vi "Teleop.vi"(10 "Match Info":T1={"Autonomous Elapsed Seconds"=0.0, "TeleOp Elapsed Seconds"=0.0, "Disabled Elapsed Seconds"=0.0, "Visited Autonomous"=FALSE, "Visited TeleOp"=FALSE, "Visited Disabled"=FALSE, "Autonomous Settings"={"Autonomous Style"=enum."Independent", "VI Refnum"=refnum}}, 11 "Call Context":T2) -> ()   [LabVIEW 2019]
doc: "This VI is called for each TeleOp packet received from the DS where the robot is not disabled. It is often used to read from the joysticks and update I/O or to update setpoints for timed control loops. It should complete and return within 20 milliseconds or it may miss DS packets."
uses:
  <vilib>/Rock Robotics/WPI/DriverStation/WPI_DriverStationDerivedRobotMode.ctl
  <vilib>/Rock Robotics/WPI/DriverStation/WPI_DriverStationMatch Info.ctl
  <vilib>/Rock Robotics/WPI/Utilities/WPI_GetSetVariantRefNum.vi
  <vilib>/Rock Robotics/Network Tables/NT Write Boolean Array.vi
  <vilib>/Rock Robotics/Network Tables/NT Write Numeric Array.vi
  <vilib>/Rock Robotics/Network Tables/NT Read Boolean.vi
  <vilib>/Rock Robotics/Network Tables/NT Read Number.vi
  Downloads/Global 2.vi
  <vilib>/Rock Robotics/Network Tables/NT Write String.vi
  <vilib>/Rock Robotics/WPI/Ultrasonic/WPI_SonarMB1010AnalogRefNum Registry Get.vi
  <vilib>/Rock Robotics/WPI/Ultrasonic/WPI_SonarMB1010AnalogGetRange.vi
  ultraG.vi
  <vilib>/functionblocks/Edge Detection/One Shot Rising with Input/One Shot Rising with Input.vi
  <vilib>/Rock Robotics/WPI/Solenoid/Deprecated/WPI_SolenoidSetBool.vi
  <vilib>/functionblocks/FB Core/FB Core.xnode
  <vilib>/functionblocks/NI_FunctionBlock Libraries.lvlib
panel:
  out "sonic":bool
  out "sensonic":bool
  in  "pegador":bool
  in  "tracao":bool
  in  "roleta":bool
  out "Matched Color Name":string
  out "Matched Color":cluster{"R":dbl, "G":dbl, "B":dbl}
  out "Color":u32(colorbox)
  out "Leitura":cluster{"R":dbl, "G":dbl, "B":dbl}
  out "Sample Slider 0":dbl(slide) scale=0.0..5.0
  out "Sample Boolean 1":bool
  out "Sample Boolean 0":bool
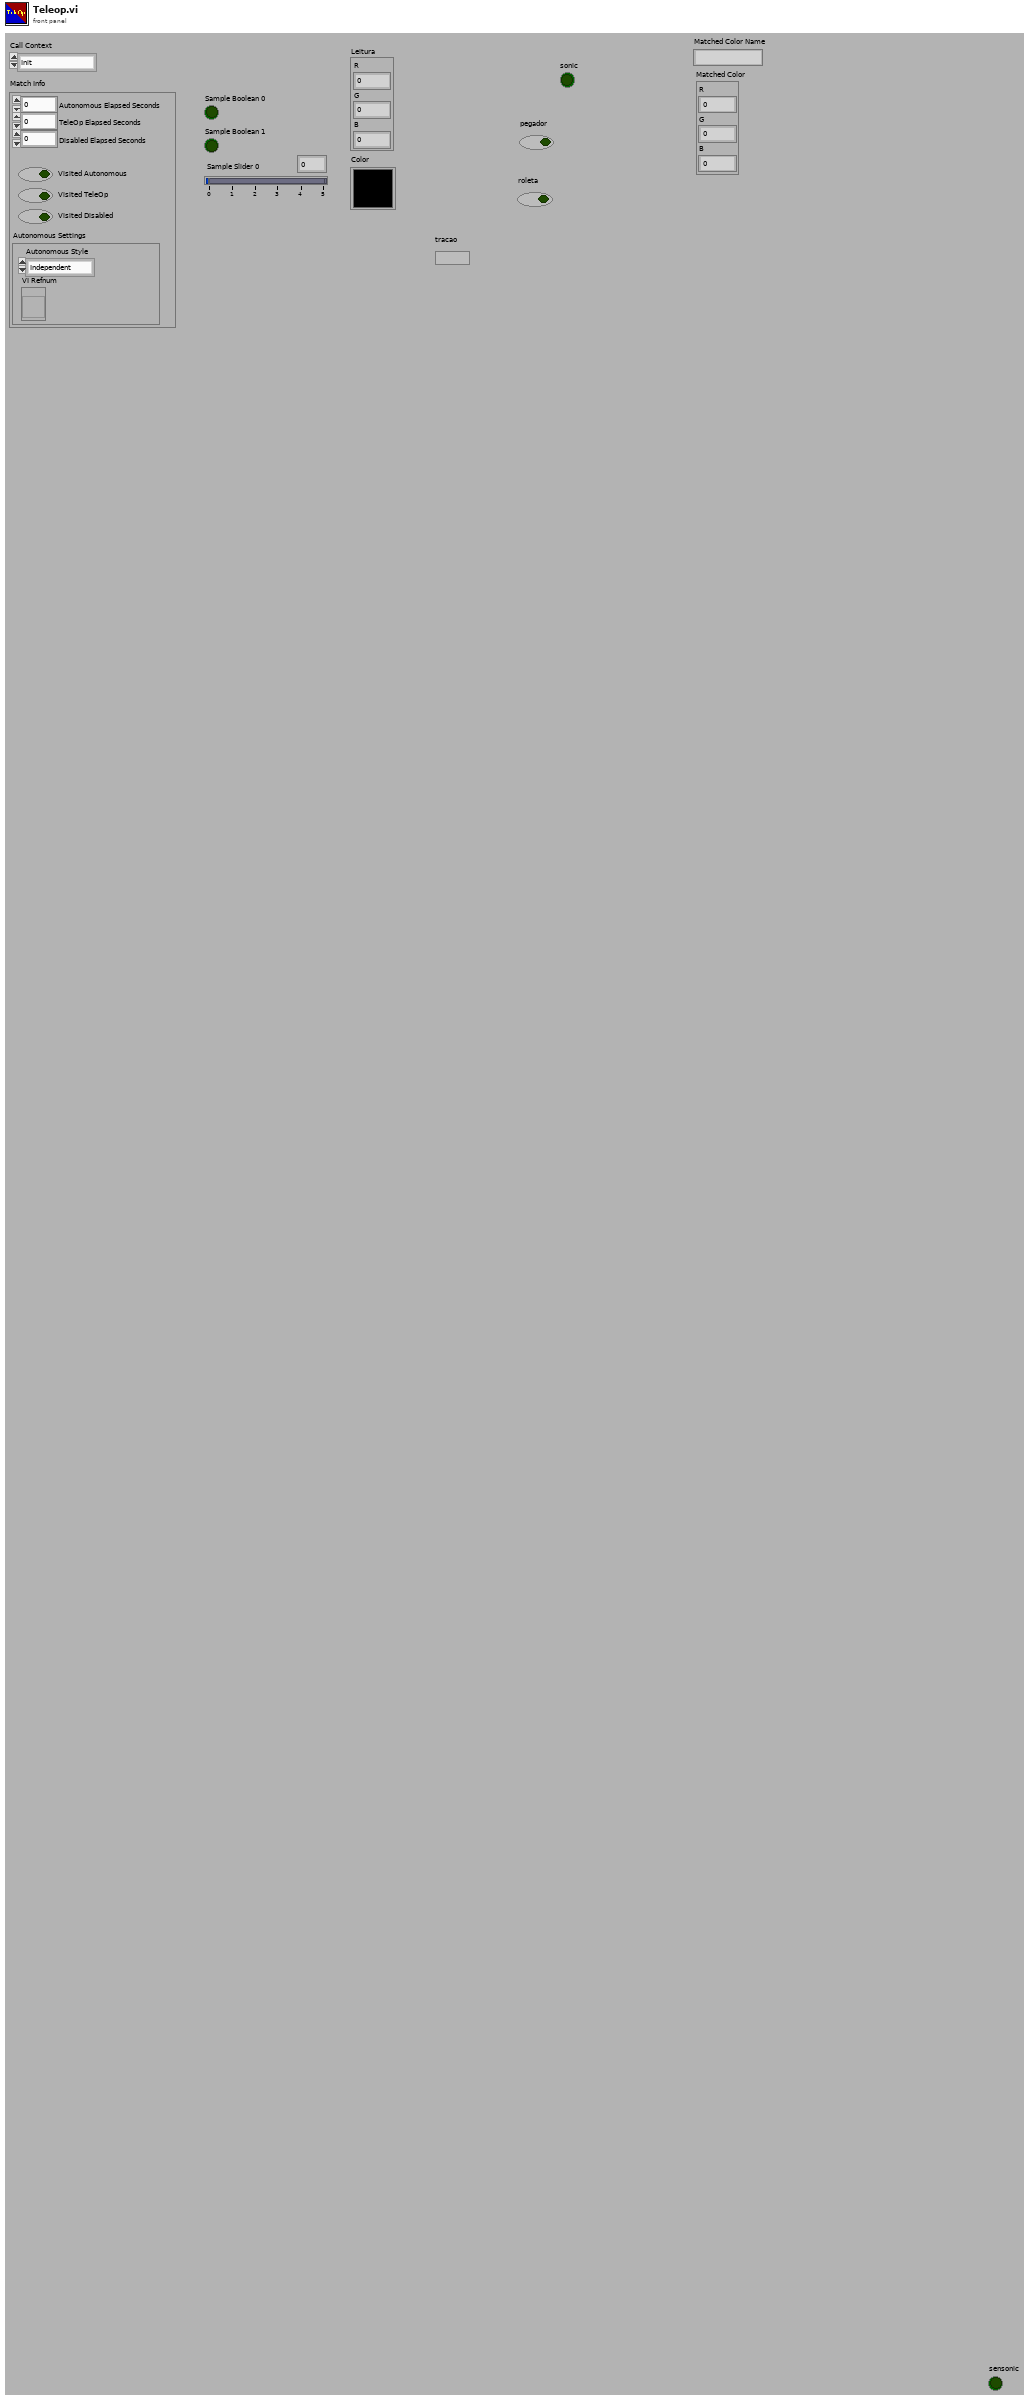
[diagram p1: front panel]
types:
  T1 = typedef "WPI_DriverStationMatch Info.ctl" = cluster{"Autonomous Elapsed Seconds":dbl, "TeleOp Elapsed Seconds":dbl, "Disabled Elapsed Seconds":dbl, "Visited Autonomous":bool, "Visited TeleOp":bool, "Visited Disabled":bool, "Autonomous Settings":cluster{"Autonomous Style":enum16{"Iterative", "Independent"}, "VI Refnum":refnum<vi>}}
  T2 = typedef "WPI_DriverStationDerivedRobotMode.ctl" = enum16{"Init", "Execute", "Stop"}
  T3 = typedef "WPI_MotorControlDeviceRef.ctl" = cluster{"DeviceStatus":errorcluster, "Type":T4, "PWM":cluster{"PWM Channel":T5, "DeadBand":T6}, "CAN":cluster{"Device Number":u8, "SetOutput VI Ref":variant, "GetOutput VI Ref":variant, "Enable VI Ref":variant, "Disable VI Ref":variant, "Data":variant}, "Invert":bool, "DIO PWM":cluster{"PWM \"Enable\" Channel":T5, "DIOChannel":T7, "PWM Rate":dbl}}
  T4 = typedef "WPI_MotorControlType.ctl" = enum16{"PWM", "CAN", "DIO PWM"}
  T5 = typedef "FPGA_DIOPWMChannel.ctl" = enum8{"PWM 0", "PWM 1", "PWM 2", "PWM 3", "PWM 4", "PWM 5", "PWM 6", "PWM 7", "PWM 8", "PWM 9", "PWM MXP 0", "PWM MXP 1", "PWM MXP 2", "PWM MXP 3", "PWM MXP 4", "PWM MXP 5", "PWM MXP 6", "PWM MXP 7", "PWM MXP 8", "PWM MXP 9", "Invalid"}
  T6 = typedef "WPI_PWMDeadband.ctl" = cluster{"Name":string, "maxPositivePwm":i32, "minPositivePwm":i32, "centerPwm":i32, "maxNegativePwm":i32, "minNegativePwm":i32, "angularRange":u16}
  T7 = typedef "FPGA_DIOChannel.ctl" = enum8{"DIO 0", "DIO 1", "DIO 2", "DIO 3", "DIO 4", "DIO 5", "DIO 6", "DIO 7", "DIO 8", "DIO 9", "DIO MXP 0", "DIO MXP 1", "DIO MXP 2", "DIO MXP 3", "DIO MXP 4", "DIO MXP 5", "DIO MXP 6", "DIO MXP 7", "DIO MXP 8", "DIO MXP 9", "DIO MXP 10", "DIO MXP 11", "DIO MXP 12", "DIO MXP 13", "DIO MXP 14", "DIO MXP 15", "SPI Port CS1", "SPI Port CS2", "SPI Port CS3", "SPI Port MISO", "SPI Port MOSI", "Invalid"}
  T8 = typedef "WPI_JoystickDevRef.ctl" = cluster{"Device":T9}
  T9 = typedef "WPI_JoystickDeviceEnum.ctl" = enum16{"USB 0", "USB 1", "USB 2", "USB 3", "USB 4", "USB 5"}
  T10 = cluster{"Axes[0]":dbl, "Axes[1]":dbl, "Axes[2]":dbl, "Axes[3]":dbl, "Axes[4]":dbl, "Axes[5]":dbl, "Axes[6]":dbl, "Axes[7]":dbl, "Axes[8]":dbl}
  T11 = cluster{"Buttons[0]":bool, "Buttons[1]":bool, "Buttons[2]":bool, "Buttons[3]":bool, "Buttons[4]":bool, "Buttons[5]":bool, "Buttons[6]":bool, "Buttons[7]":bool, "Buttons[8]":bool}
  T12 = typedef "WPI_RobotDriveDevRef.ctl" = cluster{"DevStatus":errorcluster, "Motors[]":T3[], "Square Inputs":bool, "Max Output":dbl}
  T13 = typedef "WPI_SolenoidDevRef.ctl" = cluster{"DevStatus":errorcluster, "Pneumatics Control Module":u8, "Forward Solenoid Channel":T14, "Reverse Solenoid Channel":T14}
  T14 = typedef "WPI_SolenoidChannel.ctl" = enum8{"Solenoid 0", "Solenoid 1", "Solenoid 2", "Solenoid 3", "Solenoid 4", "Solenoid 5", "Solenoid 6", "Solenoid 7", "Invalid"}
  T15 = typedef "Color Sensor V3 DevRef.ctl" = cluster{"I2CDevRef":T16}
  T16 = typedef "WPI_I2CDevRef.ctl" = cluster{"DevStatus":errorcluster, "Device Address":u8, "Handle":i32, "I2C Bus":T17}
  T17 = typedef "i2c_bus.ctl" = enum16{"I2C On-Board", "I2C MXP", "Invalid"}
  T18 = typedef "WPI_SonarMB1010AnalogDeviceRef.ctl" = cluster{"AIDeviceRef":T19, "Scaling factor (V/in)":dbl, "Average Bits":u8}
  T19 = typedef "WPI_AnalogChannelDevRef.ctl" = cluster{"DevStatus":errorcluster, "Analog Channel":T20}
  T20 = typedef "FPGA_AIChannel.ctl" = enum8{"AI 0", "AI 1", "AI 2", "AI 3", "AI MXP 0", "AI MXP 1", "AI MXP 2", "AI MXP 3", "Invalid"}
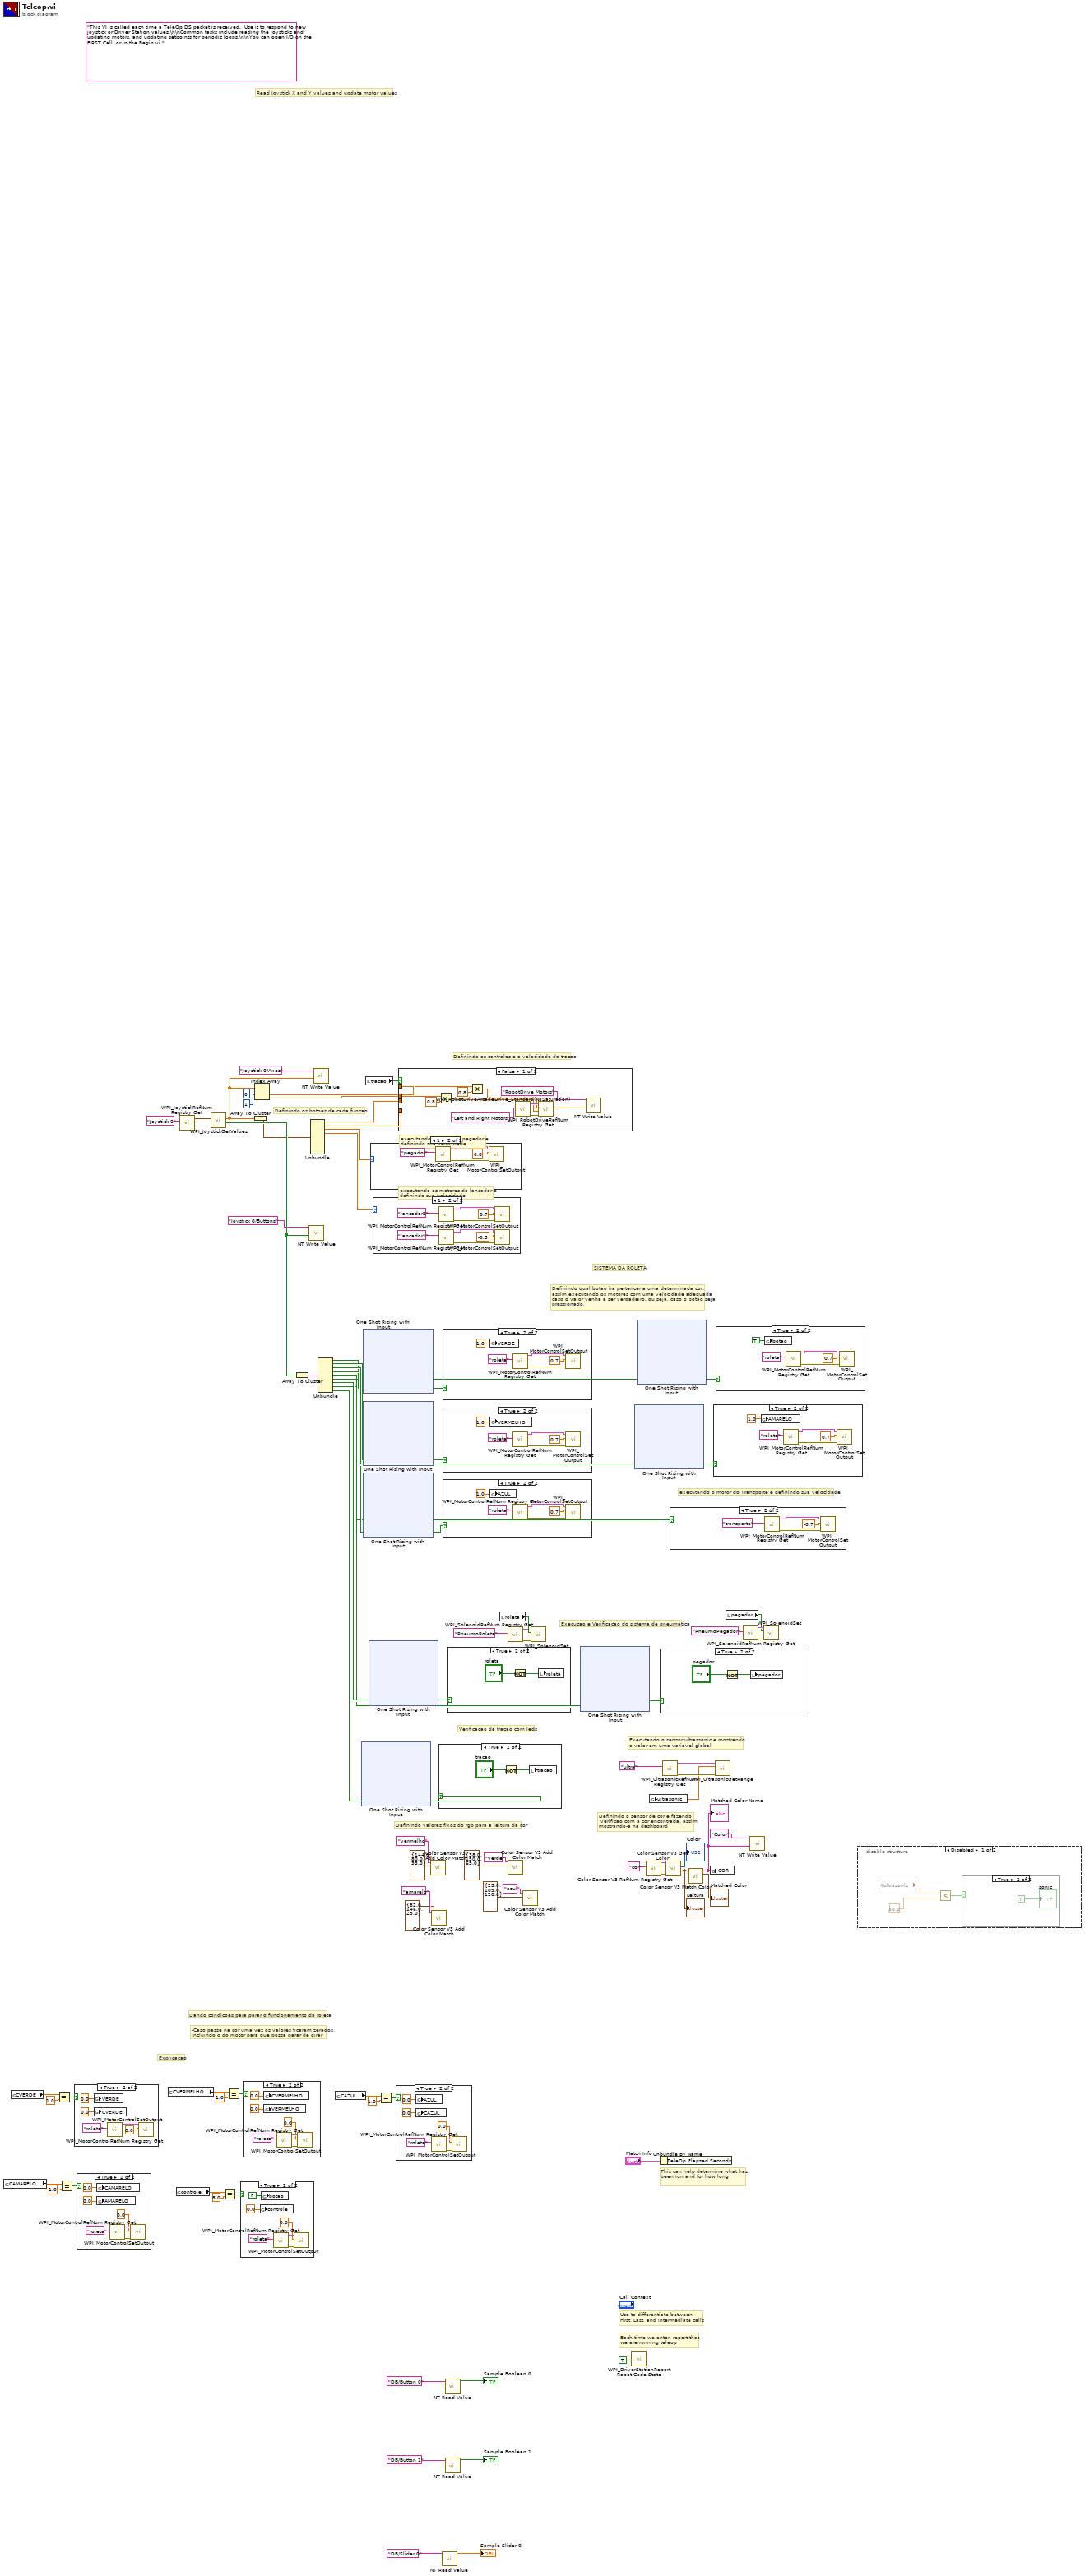
[diagram p0: block diagram]
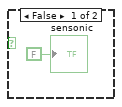
[diagram p2: hidden frame]
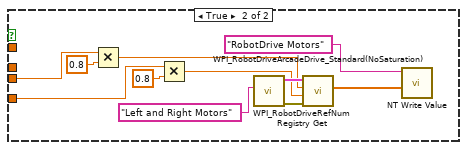
[diagram p6: hidden frame]
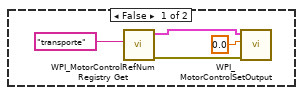
[diagram p8: hidden frame]
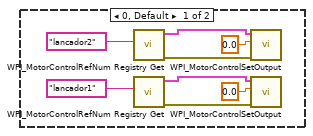
[diagram p9: hidden frame]
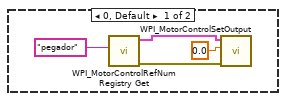
[diagram p10: hidden frame]
diagram:
  (unwired) "This VI is called each time a TeleOp DS packet is received.  Use it to respond to new joystick or Driver Station values.\n\nCommon tasks include reading the joysticks and updating motors, and updating setpoints for periodic loops.\n\nYou can open I/O on the FIRST Call, or in the Begin.vi."
  # "Explicacao"
  # "-Caso passe na cor uma vez os valores ficaram zerados,\nincluindo o do motor para que possa parar de girar"
  # "Dando condicoes para parar o funcionamento da roleta"
  # "Definindo valores fixos do rgb para a leitura da cor"
  # "Executando o sensor ultrassonic e mostrando \no valor em uma variavel global"
  # "Definindo o sensor de cor e fazendo\n verificao com a cor encontrada, assim \nmostrando-a na dashboard"
  # "Verificacao da tracao com leds"
  # "Execucao e Verificacao do sistema de pneumatica"
  # "Definindo qual botao ira pertencer a uma determinada cor,\nassim executando os motores com uma velocidade adequada \ncaso o valor venha a ser verdadeiro, ou seja, caso o botao seja\npressionado."
  # "SISTEMA DA ROLETA"
  # "executando o motor do Transporte e definindo sua velocidade"
  # "executando os motores do lancador e\ndefinindo sua velocidade"
  # "executando o motor do pegador e\ndefinindo sua velocidade"
  # "Definindo os botoes de cada funcao"
  # "Definindo os controles e a velocidade da tracao"
  # "Read Joystick X and Y values and update motor values"
  # "Each time we enter, report that\nwe are running teleop"
  # "Use to differentiate between\nFirst, Last, and Intermediate calls"
  # "This can help determine what has\nbeen run and for how long"
  n1 = global read "Global 2.vi" "CAMARELO"() -> (w38:dbl)
  n2 = global read "Global 2.vi" "CVERDE"() -> (w49:dbl)
  n3 = Equal?(x=w49, y=1.0) -> (x = y?=w47:bool)
  n4 = Equal?(x=w38, y=1.0) -> (x = y?=w40:bool)
  n5 = case shown="True" w47 {
    frame False {
    }
    frame True {
      n6 = global write "Global 2.vi" "VERDE"(0.0 ("VERDE")) -> ()
      n7 = global write "Global 2.vi" "CVERDE"(0.0 ("CVERDE")) -> ()
      n8 = call <vilib>:"WPI_MotorControlRefNum Registry Get.vi"("refnum name"="roleta") -> ("MotorControlDevRef"=w88:T3)  [unwired: 9 in, 1 out]
      n9 = call <vilib>:"WPI_MotorControlSetOutput.vi"("Output"=0.0, "MotorControlDevRef"=w88) -> ()  [unwired: 7 in, 3 out]
    }
  }
  n10 = case shown="True" w40 {
    frame False {
    }
    frame True {
      n11 = global write "Global 2.vi" "CAMARELO"(0.0 ("CAMARELO")) -> ()
      n12 = global write "Global 2.vi" "AMARELO"(0.0 ("VERDE")) -> ()
      n13 = call <vilib>:"WPI_MotorControlRefNum Registry Get.vi"("refnum name"="roleta") -> ("error out"=w92:errorcluster, "MotorControlDevRef"=w94:T3)  [unwired: 9 in]
      n14 = call <vilib>:"WPI_MotorControlSetOutput.vi"("error in (no error)"=w92, "Output"=0.0, "MotorControlDevRef"=w94) -> ()  [unwired: 6 in, 3 out]
    }
  }
  n15 = global read "Global 2.vi" "CVERMELHO"() -> (w44:dbl)
  n16 = global read "Global 2.vi" "controle"() -> (w59:dbl)
  n17 = call <vilib>:"WPI_JoystickRefNum Registry Get.vi"("refnum name"="Joystick 0") -> ("JoystickDevRef"=w83:T8)  [unwired: 1 in, 9 out]
  n18 = call <vilib>:"WPI_JoystickGetValues.vi"("JoystickDevRef"=w83) -> ("Buttons"=w63:bool[], "Axes"=w25:dbl[])  [unwired: 6 in, 3 out]
  n19 = Equal?(x=w59, y=8.0) -> (x = y?=w60:bool)
  n20 = Equal?(x=w44, y=1.0) -> (x = y?=w46:bool)
  n21 = case shown="True" w60 {
    frame False {
    }
    frame True {
      n22 = global write "Global 2.vi" "controle"(0.0 ("controle")) -> ()
      n23 = global write "Global 2.vi" "botão"(FALSE ("botão")) -> ()
      n24 = call <vilib>:"WPI_MotorControlRefNum Registry Get.vi"("refnum name"="roleta") -> ("error out"=w98:errorcluster, "MotorControlDevRef"=w100:T3)  [unwired: 9 in]
      n25 = call <vilib>:"WPI_MotorControlSetOutput.vi"("error in (no error)"=w98, "Output"=0.0, "MotorControlDevRef"=w100) -> ()  [unwired: 6 in, 3 out]
    }
  }
  n26 = case shown="True" w46 {
    frame False {
    }
    frame True {
      n27 = global write "Global 2.vi" "CVERMELHO"(0.0 ("CVERMELHO")) -> ()
      n28 = global write "Global 2.vi" "VERMELHO"(0.0 ("VERDE")) -> ()
      n29 = call <vilib>:"WPI_MotorControlRefNum Registry Get.vi"("refnum name"="roleta") -> ("error out"=w104:errorcluster, "MotorControlDevRef"=w106:T3)  [unwired: 9 in]
      n30 = call <vilib>:"WPI_MotorControlSetOutput.vi"("error in (no error)"=w104, "Output"=0.0, "MotorControlDevRef"=w106) -> ()  [unwired: 6 in, 3 out]
    }
  }
  n31 = Array To Cluster(array=w25) -> (cluster=w28:T10)
  n32 = Index Array(array=w25, index #1=0 ("index"), index #2=1 ("index")) -> (element #1=w11:dbl, element #2=w10:dbl)
  n33 = Array To Cluster(array=w63) -> (cluster=w62:T11)
  n34 = call-poly <vilib>:"NT Write Value.vi"("Boolean Array"=w63, "Name"="Joystick 0/Buttons") -> ()  [unwired: 9 in, 1 out]
  n35 = Unbundle(w28) -> ("Axes[0]"=w12:dbl, "Axes[1]"=w13:dbl, "Axes[2]"=w27:dbl, "Axes[3]"=w23:dbl)  [unwired: 5 out]
  n36 = call-poly <vilib>:"NT Write Value.vi"("Numeric Array"=w25, "Name"="Joystick 0/Axes") -> ()  [unwired: 9 in, 1 out]
  n37 = Unbundle(w62) -> ("Buttons[0]"=w26:bool, "Buttons[1]"=w53:bool, "Buttons[2]"=w50:bool, "Buttons[3]"=w52:bool, "Buttons[4]"=w14:bool, "Buttons[5]"=w37:bool, "Buttons[6]"=w17:bool, "Buttons[7]"=w1:bool, "Buttons[8]"=w8:bool)
  n38 = global read "Global 2.vi" "CAZUL"() -> (w43:dbl)
  n39 = xnode "One Shot Rising with Input"("input"=w8) -> ("output"=w9:bool)  [unwired: 1 in, 1 out]
  n40 = xnode "One Shot Rising with Input"("input"=w26) -> ("output"=w24:bool)  [unwired: 1 in, 1 out]
  n41 = xnode "One Shot Rising with Input"("input"=w53) -> ("output"=w55:bool)  [unwired: 1 in, 1 out]
  n42 = xnode "One Shot Rising with Input"("input"=w50) -> ("output"=w51:bool)  [unwired: 1 in, 1 out]
  n43 = local read "tracao"() -> (w7:bool)
  n44 = xnode "One Shot Rising with Input"("input"=w17) -> ("output"=w18:bool)  [unwired: 1 in, 1 out]
  n45 = case shown="1" w27 {
    frame 0, Default {
      n46 = call <vilib>:"WPI_MotorControlRefNum Registry Get.vi"("refnum name"="pegador") -> ("error out"=w111:errorcluster, "MotorControlDevRef"=w112:T3)  [unwired: 9 in]
      n47 = call <vilib>:"WPI_MotorControlSetOutput.vi"("error in (no error)"=w111, "Output"=0.0, "MotorControlDevRef"=w112) -> ()  [unwired: 6 in, 3 out]
    }
    frame 1 {
      n48 = call <vilib>:"WPI_MotorControlRefNum Registry Get.vi"("refnum name"="pegador") -> ("error out"=w115:errorcluster, "MotorControlDevRef"=w116:T3)  [unwired: 9 in]
      n49 = call <vilib>:"WPI_MotorControlSetOutput.vi"("error in (no error)"=w115, "Output"=0.8, "MotorControlDevRef"=w116) -> ()  [unwired: 6 in, 3 out]
    }
  }
  n50 = case shown="1" w23 {
    frame 0, Default {
      n51 = call <vilib>:"WPI_MotorControlRefNum Registry Get.vi"("refnum name"="lancador2") -> ("error out"=w123:errorcluster, "MotorControlDevRef"=w124:T3)  [unwired: 9 in]
      n52 = call <vilib>:"WPI_MotorControlRefNum Registry Get.vi"("refnum name"="lancador1") -> ("error out"=w121:errorcluster, "MotorControlDevRef"=w122:T3)  [unwired: 9 in]
      n53 = call <vilib>:"WPI_MotorControlSetOutput.vi"("error in (no error)"=w123, "Output"=0.0, "MotorControlDevRef"=w124) -> ()  [unwired: 6 in, 3 out]
      n54 = call <vilib>:"WPI_MotorControlSetOutput.vi"("error in (no error)"=w121, "Output"=0.0, "MotorControlDevRef"=w122) -> ()  [unwired: 6 in, 3 out]
    }
    frame 1 {
      n55 = call <vilib>:"WPI_MotorControlRefNum Registry Get.vi"("refnum name"="lancador2") -> ("error out"=w131:errorcluster, "MotorControlDevRef"=w132:T3)  [unwired: 9 in]
      n56 = call <vilib>:"WPI_MotorControlRefNum Registry Get.vi"("refnum name"="lancador1") -> ("error out"=w129:errorcluster, "MotorControlDevRef"=w130:T3)  [unwired: 9 in]
      n57 = call <vilib>:"WPI_MotorControlSetOutput.vi"("error in (no error)"=w131, "Output"=0.7, "MotorControlDevRef"=w132) -> ()  [unwired: 6 in, 3 out]
      n58 = call <vilib>:"WPI_MotorControlSetOutput.vi"("error in (no error)"=w129, "Output"=-0.5, "MotorControlDevRef"=w130) -> ()  [unwired: 6 in, 3 out]
    }
  }
  n59 = Equal?(x=w43, y=1.0) -> (x = y?=w41:bool)
  n60 = case shown="True" w41 {
    frame False {
    }
    frame True {
      n61 = global write "Global 2.vi" "AZUL"(0.0 ("VERDE")) -> ()
      n62 = global write "Global 2.vi" "CAZUL"(0.0 ("CAZUL")) -> ()
      n63 = call <vilib>:"WPI_MotorControlRefNum Registry Get.vi"("refnum name"="roleta") -> ("error out"=w134:errorcluster, "MotorControlDevRef"=w136:T3)  [unwired: 9 in]
      n64 = call <vilib>:"WPI_MotorControlSetOutput.vi"("error in (no error)"=w134, "Output"=0.0, "MotorControlDevRef"=w136) -> ()  [unwired: 6 in, 3 out]
    }
  }
  n65 = case shown="False" w7 {
    tunnel: w13 -> [_ w151]
    tunnel: w12 -> [_ w154]
    tunnel: w11 -> [w139 _]
    tunnel: w10 -> [w143 _]
    frame False {
      n66 = Multiply(x=w143, y=0.8) -> (x*y=w144:dbl)
      n67 = Multiply(x=w139, y=0.8) -> (x*y=w140:dbl)
      n68 = call <vilib>:"WPI_RobotDriveRefNum Registry Get.vi"("refnum name"="Left and Right Motors") -> ("error out"=w146:errorcluster, "RobotDriveDevRef"=w147:T12)  [unwired: 1 in, 8 out]
      n69 = call <vilib>:"WPI_RobotDriveArcadeDrive_Standard(NoSaturation).vi"("error in (no error)"=w146, "Y axis value"=w144, "X axis value"=w140, "RobotDriveDevRef"=w147) -> ("Motor Values"=w145:dbl[])  [unwired: 7 out]
      n70 = call-poly <vilib>:"NT Write Value.vi"("Numeric Array"=w145, "Name"="RobotDrive Motors") -> ()  [unwired: 9 in, 1 out]
    }
    frame True {
      n71 = Multiply(x=w154, y=0.8) -> (x*y=w155:dbl)
      n72 = Multiply(x=w151, y=0.8) -> (x*y=w152:dbl)
      n73 = call <vilib>:"WPI_RobotDriveRefNum Registry Get.vi"("refnum name"="Left and Right Motors") -> ("error out"=w156:errorcluster, "RobotDriveDevRef"=w159:T12)  [unwired: 1 in, 8 out]
      n74 = call <vilib>:"WPI_RobotDriveArcadeDrive_Standard(NoSaturation).vi"("error in (no error)"=w156, "Y axis value"=w152, "X axis value"=w155, "RobotDriveDevRef"=w159) -> ("Motor Values"=w158:dbl[])  [unwired: 7 out]
      n75 = call-poly <vilib>:"NT Write Value.vi"("Numeric Array"=w158, "Name"="RobotDrive Motors") -> ()  [unwired: 9 in, 1 out]
    }
  }
  n76 = call <vilib>:"Color Sensor V3 Add Color Match.vi"("Color"=cluster{"R":dbl, "G":dbl, "B":dbl} {"R"=144.0, "G"=80.0, "B"=33.0}, "Name"="vermelho") -> ()  [unwired: 10 in]
  n77 = call <vilib>:"Color Sensor V3 Add Color Match.vi"("Color"=cluster{"R":dbl, "G":dbl, "B":dbl} {"R"=82.0, "G"=146.0, "B"=25.0}, "Name"="amarelo") -> ()  [unwired: 10 in]
  n78 = case shown="True" w9 {
    frame False {
    }
    frame True {
      n79 = Not(x="tracao") -> (.not. x?=w162:bool)
      n80 = local write "tracao"(w162) -> ()
    }
  }
  n81 = call-poly <vilib>:"NT Read Value.vi"("Name"="DB/Slider 0" ("refnum name")) -> ("Numeric"=→"Sample Slider 0":dbl)  [unwired: 9 in, 1 out]
  n82 = case shown="True" w24 {
    frame False {
    }
    frame True {
      n83 = global write "Global 2.vi" "VERDE"(1.0 ("VERDE")) -> ()
      n84 = call <vilib>:"WPI_MotorControlRefNum Registry Get.vi"("refnum name"="roleta") -> ("error out"=w166:errorcluster, "MotorControlDevRef"=w165:T3)  [unwired: 9 in]
      n85 = call <vilib>:"WPI_MotorControlSetOutput.vi"("error in (no error)"=w166, "Output"=0.7, "MotorControlDevRef"=w165) -> ()  [unwired: 6 in, 3 out]
    }
  }
  n86 = case shown="True" w55 {
    frame False {
    }
    frame True {
      n87 = global write "Global 2.vi" "VERMELHO"(1.0 ("VERMELHO")) -> ()
      n88 = call <vilib>:"WPI_MotorControlRefNum Registry Get.vi"("refnum name"="roleta") -> ("error out"=w172:errorcluster, "MotorControlDevRef"=w171:T3)  [unwired: 9 in]
      n89 = call <vilib>:"WPI_MotorControlSetOutput.vi"("error in (no error)"=w172, "Output"=0.7, "MotorControlDevRef"=w171) -> ()  [unwired: 6 in, 3 out]
    }
  }
  n90 = case shown="True" w51 {
    frame False {
    }
    frame True {
      n91 = global write "Global 2.vi" "AZUL"(1.0 ("AZUL")) -> ()
      n92 = call <vilib>:"WPI_MotorControlRefNum Registry Get.vi"("refnum name"="roleta") -> ("error out"=w176:errorcluster, "MotorControlDevRef"=w175:T3)  [unwired: 9 in]
      n93 = call <vilib>:"WPI_MotorControlSetOutput.vi"("error in (no error)"=w176, "Output"=0.7, "MotorControlDevRef"=w175) -> ()  [unwired: 6 in, 3 out]
    }
  }
  n94 = call-poly <vilib>:"NT Read Value.vi"("Name"="DB/Button 0" ("refnum name")) -> ("Boolean"=→"Sample Boolean 0":bool)  [unwired: 9 in, 1 out]
  n95 = call-poly <vilib>:"NT Read Value.vi"("Name"="DB/Button 1" ("refnum name")) -> ("Boolean"=→"Sample Boolean 1":bool)  [unwired: 9 in, 1 out]
  n96 = case shown="True" w18 {
    frame False {
    }
    frame True {
      n97 = Not(x="roleta") -> (.not. x?=w179:bool)
      n98 = local write "roleta"(w179) -> ()
    }
  }
  n99 = local read "roleta"() -> (w22:bool)
  n100 = call <vilib>:"WPI_SolenoidRefNum Registry Get.vi"("refnum name"="PneumoRoleta") -> ("error out"=w19:errorcluster, "SolenoidDevRef"=w20:T13)  [unwired: 9 in]
  n101 = call <vilib>:"Color Sensor V3 Add Color Match.vi"("Color"=cluster{"R":dbl, "G":dbl, "B":dbl} {"R"=38.0, "G"=150.0, "B"=65.0}, "Name"="verde") -> ()  [unwired: 10 in]
  n102 = call <vilib>:"Color Sensor V3 Add Color Match.vi"("Color"=cluster{"R":dbl, "G":dbl, "B":dbl} {"R"=25.0, "G"=105.0, "B"=120.0}, "Name"="azul") -> ()  [unwired: 10 in]
  n103 = call-poly <vilib>:"WPI_SolenoidSet.vi"("error in (no error)"=w19, "Value"=w22, "SolenoidDevRef"=w20) -> ()  [unwired: 7 in, 2 out]
  n104 = xnode "One Shot Rising with Input"("input"=w1) -> ("output"=w2:bool)  [unwired: 1 in, 1 out]
  n105 = call <vilib>:"WPI_DriverStationReport Robot Code State.vi"("TeleOp"=TRUE ("Autonomous")) -> ()  [unwired: 10 in, 1 out]
  n106 = xnode "One Shot Rising with Input"("input"=w52) -> ("output"=w54:bool)  [unwired: 1 in, 1 out]
  n107 = xnode "One Shot Rising with Input"("input"=w37) -> ("output"=w61:bool)  [unwired: 1 in, 1 out]
  n108 = call <vilib>:"Color Sensor V3 RefNum Registry Get.vi"("refnum name"="cor") -> ("error out"=w73:errorcluster, "ColorSensorDevRef"=w72:T15)  [unwired: 9 in]
  n109 = case shown="True" w2 {
    frame False {
    }
    frame True {
      n110 = Not(x="pegador") -> (.not. x?=w180:bool)
      n111 = local write "pegador"(w180) -> ()
    }
  }
  n112 = Unbundle By Name("Match Info") -> ()  [unwired: 1 out]
  n113 = call-poly <vilib>:"WPI_UltrasonicRefNum Registry Get.vi"("refnum name"="ultra") -> ("error out"=w32:errorcluster, "SonarMB1010AnalogDevRef"=w31:T18)  [unwired: 9 in]
  n114 = call <vilib>:"Color Sensor V3 Get Color.vi"("error in (no error)"=w73, "ColorSensorDevRef"=w72) -> ("Normalized Color"=w65:cluster{"R":dbl, "G":dbl, "B":dbl}, "Color"=→"Color":u32)  [unwired: 6 in, 2 out]
  "Leitura" <- w65
  n115 = case shown="True" w14 {
    frame False {
      n116 = call <vilib>:"WPI_MotorControlRefNum Registry Get.vi"("refnum name"="transporte") -> ("error out"=w183:errorcluster, "MotorControlDevRef"=w184:T3)  [unwired: 9 in]
      n117 = call <vilib>:"WPI_MotorControlSetOutput.vi"("error in (no error)"=w183, "Output"=0.0 ("Motor Output"), "MotorControlDevRef"=w184) -> ()  [unwired: 6 in, 3 out]
    }
    frame True {
      n118 = call <vilib>:"WPI_MotorControlRefNum Registry Get.vi"("refnum name"="transporte") -> ("error out"=w188:errorcluster, "MotorControlDevRef"=w189:T3)  [unwired: 9 in]
      n119 = call <vilib>:"WPI_MotorControlSetOutput.vi"("error in (no error)"=w188, "Output"=-0.7, "MotorControlDevRef"=w189) -> ()  [unwired: 6 in, 3 out]
    }
  }
  n120 = call <vilib>:"Color Sensor V3 Match Color.vi"("Measured Color"=w65) -> ("Matched Color"=→"Matched Color":cluster{"R":dbl, "G":dbl, "B":dbl}, "Matched Color Name"=w57:string)  [unwired: 8 in, 1 out]
  "Matched Color Name" <- w57
  n121 = global write "Global 2.vi" "COR"(w57) -> ()
  n122 = case shown="True" w54 {
    frame False {
    }
    frame True {
      n123 = global write "Global 2.vi" "AMARELO"(1.0 ("AMARELO")) -> ()
      n124 = call <vilib>:"WPI_MotorControlRefNum Registry Get.vi"("refnum name"="roleta") -> ("error out"=w193:errorcluster, "MotorControlDevRef"=w192:T3)  [unwired: 9 in]
      n125 = call <vilib>:"WPI_MotorControlSetOutput.vi"("error in (no error)"=w193, "Output"=0.7, "MotorControlDevRef"=w192) -> ()  [unwired: 6 in, 3 out]
    }
  }
  n126 = call-poly <vilib>:"WPI_UltrasonicGetRange.vi"("error in"=w32, "SonarMB1010AnalogDevRef"=w31) -> ("Distance"=w29:dbl)  [unwired: 7 in, 2 out]
  n127 = global write "ultraG.vi" "ultrasonic"(w29) -> ()
  n128 = case shown="True" w61 {
    frame False {
    }
    frame True {
      n129 = global write "Global 2.vi" "botão"(TRUE ("botão")) -> ()
      n130 = call <vilib>:"WPI_MotorControlRefNum Registry Get.vi"("refnum name"="roleta") -> ("error out"=w196:errorcluster, "MotorControlDevRef"=w198:T3)  [unwired: 9 in]
      n131 = call <vilib>:"WPI_MotorControlSetOutput.vi"("error in (no error)"=w196, "Output"=0.7, "MotorControlDevRef"=w198) -> ()  [unwired: 6 in, 3 out]
    }
  }
  n132 = local read "pegador"() -> (w3:bool)
  n133 = call <vilib>:"WPI_SolenoidRefNum Registry Get.vi"("refnum name"="PneumoPegador") -> ("error out"=w4:errorcluster, "SolenoidDevRef"=w5:T13)  [unwired: 9 in]
  n134 = call-poly <vilib>:"NT Write Value.vi"("String"=w57, "Name"="Color") -> ()  [unwired: 9 in, 1 out]
  n135 = call-poly <vilib>:"WPI_SolenoidSet.vi"("error in (no error)"=w4, "Value"=w3, "SolenoidDevRef"=w5) -> ()  [unwired: 7 in, 2 out]
  n136 = disable-structure shown="Disabled" {
    frame Disabled {
      n137 = global read "ultraG.vi" "ultrasonic"() -> (w201:dbl)
      n138 = Less?(x=w201, y=30.0) -> (x < y?=w202:bool)
      n139 = case shown="True" w202 {
        frame False {
          "sensonic" <- FALSE ("sensonic")
        }
        frame True {
          "sonic" <- TRUE ("sonic")
        }
      }
    }
    frame Enabled {
    }
  }
